vi "AB_API Resolve References.vi"(8 "error in (no error)":errorcluster, 10 "Project Refnum":refnum<vi>, 11 "TargetItem Refnum":refnum<vi>) -> (0 "error out":errorcluster, 1 "TargetItem reference":refnum<vi>, 2 "project path null?":bool, 3 "using My Computer?":bool)   [LabVIEW 2020]
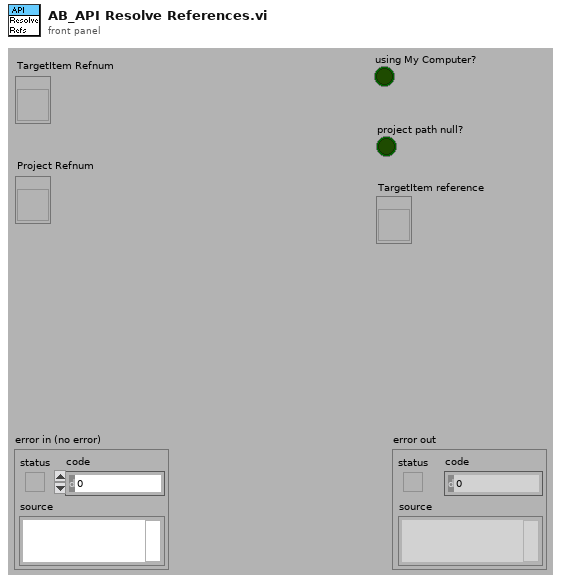
[diagram p1: front panel]
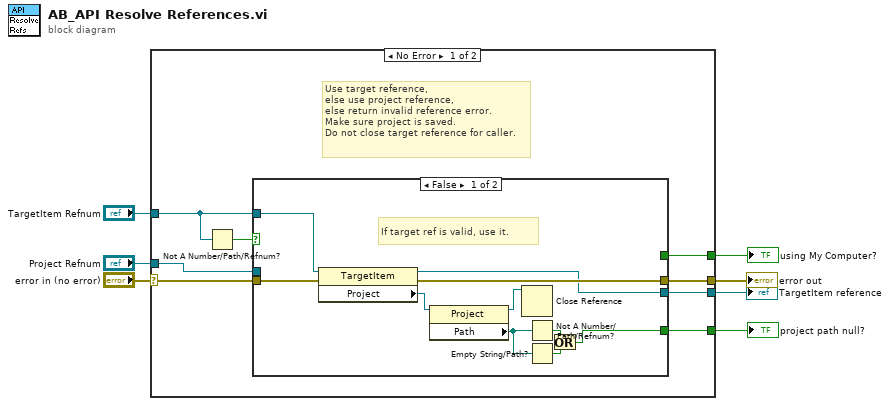
[diagram p0: block diagram]
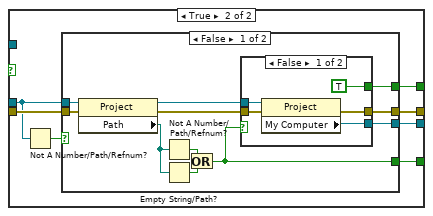
[diagram p2: hidden frame]
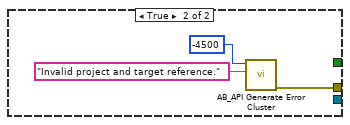
[diagram p4: hidden frame]
diagram:
  n1 = case shown="No Error" "error in (no error)" {
    selector: "error in (no error)" -> [w13 w53]
    tunnel: [w14 w53] -> w6
    tunnel: "Project Refnum" -> [w11 _]
    tunnel: "TargetItem Refnum" -> [w12 _]
    tunnel: [w10 _] -> w3
    tunnel: [w9 _] -> w2
    tunnel: [w8 _] -> w1
    frame No Error {
      # "Use target reference,\nelse use project reference,\nelse return invalid reference error.\nMake sure project is saved.\nDo not close target reference for caller."
      n2 = Not A Number/Path/Refnum?(number/path/refnum=w12) -> (NaN/Path/Refnum?=w15:bool)
      n3 = case shown="False" w15 {
        tunnel: [w22 w32] -> w8
        tunnel: [w23 w31] -> w14
        tunnel: w11 -> [_ w28]
        tunnel: w12 -> [w16 _]
        tunnel: w13 -> [w25 w30]
        tunnel: [w17 w29] -> w9
        tunnel: [_ w26] -> w10
        frame False {
          # "If target ref is valid, use it."
          n4 = property class="TargetItem"(reference=w16, error in=w25) -> (reference out=w22:refnum<vi>, error out=w23:errorcluster, "Project"=w24:refnum<vi>)
          n5 = property class="Project"(reference=w24) -> (reference out=w21:refnum<vi>, "Path"=w18:path)  [unwired: 1 in, 1 out]
          n6 = Close Reference(reference=w21) -> ()  [unwired: 1 in, 1 out]
          n7 = Not A Number/Path/Refnum?(number/path/refnum=w18) -> (NaN/Path/Refnum?=w20:bool)
          n8 = Empty String/Path?(string/path=w18) -> (empty?=w19:bool)
          n9 = Or(x=w20, y=w19) -> (x .or. y?=w17:bool)
        }
        frame True {
          n10 = Not A Number/Path/Refnum?(number/path/refnum=w28) -> (NaN/Path/Refnum?=w27:bool)
          n11 = case shown="False" w27 {
            tunnel: [w43 _] -> w32
            tunnel: [w42 w50] -> w31
            tunnel: w30 -> [w40 _]
            tunnel: [w35 _] -> w29
            tunnel: w28 -> [w34 _]
            tunnel: [w33 _] -> w26
            frame False {
              n12 = property class="Project"(reference=w34, error in=w40) -> (reference out=w41:refnum<vi>, error out=w39:errorcluster, "Path"=w38:path)
              n13 = Not A Number/Path/Refnum?(number/path/refnum=w38) -> (NaN/Path/Refnum?=w37:bool)
              n14 = Empty String/Path?(string/path=w38) -> (empty?=w36:bool)
              n15 = Or(x=w37, y=w36) -> (x .or. y?=w35:bool)
              n16 = case shown="False" w35 {
                tunnel: [w48 _] -> w43
                tunnel: [w47 w49] -> w42
                tunnel: w41 -> [w46 _]
                tunnel: w39 -> [w45 w49]
                tunnel: [TRUE _] -> w33
                frame False {
                  n17 = property class="Project"(reference=w46, error in=w45) -> (error out=w47:errorcluster, "My Computer"=w48:refnum<vi>)  [unwired: 1 out]
                }
                frame True {
                }
              }
            }
            frame True {
              n18 = call <vilib>:"AB_API Generate Error Cluster.vi"("Additional Message"="Invalid project and target reference.", "Code"=-4500) -> ("error out"=w50:errorcluster)  [unwired: 2 in, 7 out]
            }
          }
        }
      }
    }
    frame Error {
    }
  }
  "error out" <- w6
  "using My Computer?" <- w3
  "project path null?" <- w2
  "TargetItem reference" <- w1
